vi "Pump Global Variables.vi"() -> ()   [LabVIEW 2020]
panel:
  in  "Units 2":string(combo)="mm"
  in  "Incr/Decr Time (S)":dbl
  in  "Pump Direction":string(combo)="inf"
  in  "Diameter (mm)":dbl=0.1 min=0.1 max=50.0
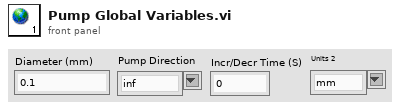
[diagram p1: front panel]
diagram:
